vi "Read Code.vi"(8 "error in (no error)":errorcluster, 11 "SimpleEvent in":refnum<class "SimpleEvent.lvclass">) -> (0 "error out":errorcluster, 2 "Code":dbl, 3 "SimpleEvent out":refnum<class "SimpleEvent.lvclass">)   [LabVIEW 2012, in "SimpleEvent.lvclass"]
uses:
  SimpleEvent.lvclass
  SimpleEvent.lvclass/SimpleEvent.ctl
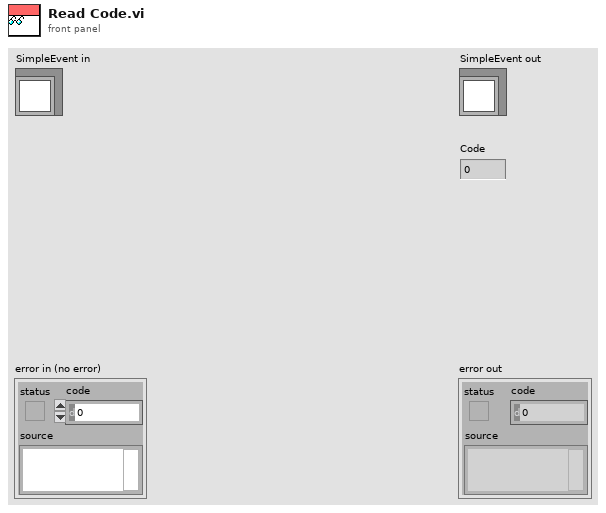
[diagram p1: front panel]
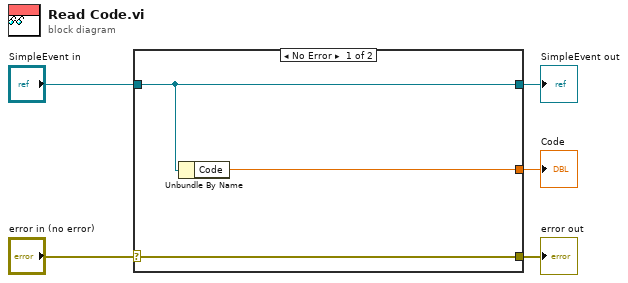
[diagram p0: block diagram]
diagram:
  n1 = case shown="No Error" "error in (no error)" {
    selector: "error in (no error)" -> [w8 w9]
    tunnel: [w8 w9] -> w4
    tunnel: [w7 w10] -> w2
    tunnel: "SimpleEvent in" -> [w7 w10]
    tunnel: [w6 _] -> w1
    frame No Error {
      n2 = Unbundle By Name(w7) -> ("Code"=w6:dbl)
    }
    frame Error {
    }
  }
  "error out" <- w4
  "SimpleEvent out" <- w2
  "Code" <- w1
